vi "Robot Main.vi"() -> ()   [LabVIEW 2014]
doc: "This VI implements the framework and scheduler for your robotics program. It should not be necessary to modify the framework. You are expected to add your code to the VIs called from Robot Main - the ones located in the Team Code folder within the project."
uses:
  <vilib>/Rock Robotics/WPI/Camera/WPI_CameraImageSize.ctl
  Robot Global Data.vi
panel:
  out "Trace Buffer Size":i32
  in  "Image Size":T1=enum."320x240"
  in  "Enable Vision":bool
  in  "Finish":bool
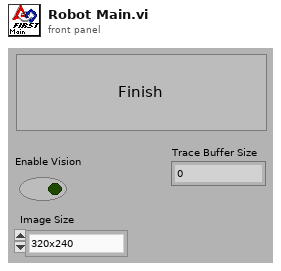
[diagram p1: front panel]
types:
  T1 = typedef "WPI_CameraImageSize.ctl" = enum16{"640x480", "320x240", "160x120", "Custom"}
  T2 = typedef "WPI_DriverStationMatch Info.ctl" = cluster{"Autonomous Elapsed Seconds":dbl, "TeleOp Elapsed Seconds":dbl, "Disabled Elapsed Seconds":dbl, "Visited Autonomous":bool, "Visited TeleOp":bool, "Visited Disabled":bool, "Autonomous Settings":cluster{"Autonomous Style":enum16{"Iterative", "Independent"}, "VI Refnum":refnum<vi>}}
  T3 = typedef "WPI_DriverStationDerivedRobotMode.ctl" = enum16{"Init", "Execute", "Stop"}
  T4 = typedef "WPI_DriverStationRobotMode2.ctl" = enum16{"Autonomous Disabled", "Autonomous Enabled", "Teleop Disabled", "Teleop Enabled", "Disconnected", "Finish", "Test Disabled", "Test Enabled", "Emergency Stopped"}
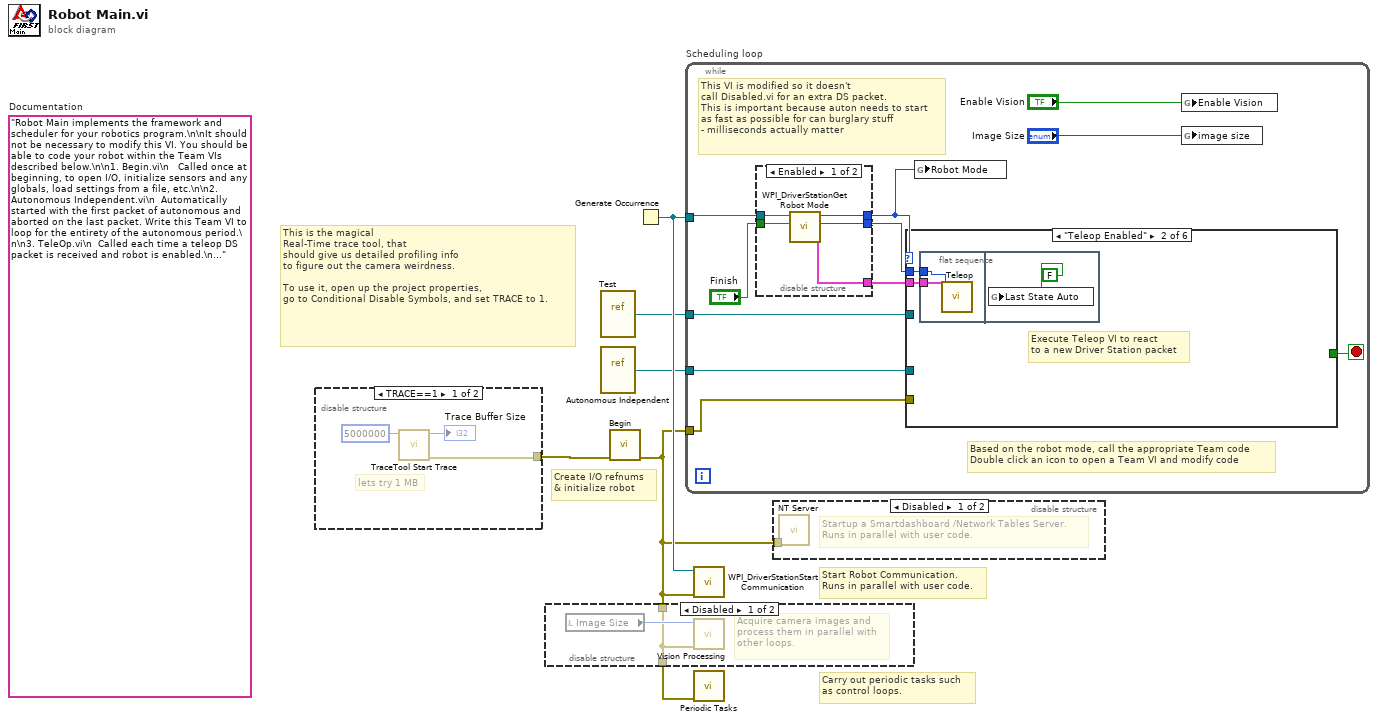
[diagram p0: block diagram]
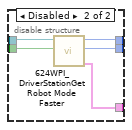
[diagram p5: hidden frame]
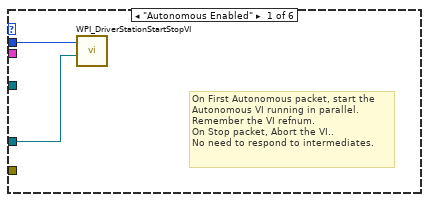
[diagram p6: hidden frame]
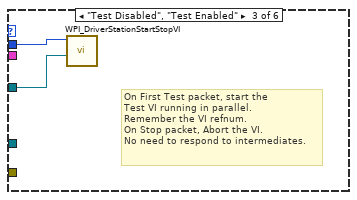
[diagram p7: hidden frame]
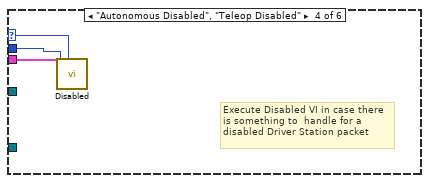
[diagram p8: hidden frame]
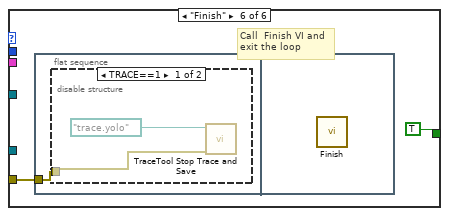
[diagram p10: hidden frame]
diagram:
  (unwired) "Robot Main implements the framework and scheduler for your robotics program.\n\nIt should not be necessary to modify this VI. You should be able to code your robot within the Team VIs described below.\n\n1. Begin.vi\n   Called once at beginning, to open I/O, initialize sensors and any globals, load settings from a file, etc.\n\n2. Autonomous Independent.vi\n  Automatically started with the first packet of autonomous and aborted on the last packet. Write this Team VI to loop for the entirety of the autonomous period.\n\n3. TeleOp.vi\n  Called each time a teleop DS packet is received and robot is enabled.\n\n4. Disabled.vi\n  Called each time a packet is received and the robot is disabled.\n\n5. Test.vi\n  Called Automatically started with the first test packet and aborted on the last. Modify this VI to carry out robot and sensor validation tests.\n\n6. Vision.vi\n  A parallel loop that acquires and processes camera images.\n\n7. PeriodicTasks.vi\n  Parallel loops running at user-defined rates.\n\n8. Finish.vi\n  Called before exiting, so you can save data, clean up I/O, etc.\n"  # Documentation
  # "Create I/O refnums\n& initialize robot"
  # "This is the magical\nReal-Time trace tool, that\nshould give us detailed profiling info \nto figure out the camera weirdness.\n\nTo use it, open up the project properties,\ngo to Conditional Disable Symbols, and set TRACE to 1."
  # "Carry out periodic tasks such\nas control loops."
  # "Start Robot Communication.\nRuns in parallel with user code."
  n1 = disable-structure shown="TRACE==1" {
    disable-tunnel: [w9 _] -> w1
    frame condition #0 {
      # "lets try 1 MB"
      n2 = call <vilib>:"TraceTool Start Trace.vi"("Buffer Size (250000 bytes)"=5000000) -> ("error out"=w9:errorcluster, "Actual Buffer Size"=→"Trace Buffer Size":i32)  [unwired: 9 in]
    }
    frame condition #1 (active) {
    }
  }
  n3 = vi-ref "Test.vi"() -> (w4:refnum<vi>)
  n4 = vi-ref "Autonomous Independent.vi"() -> (w5:refnum<vi>)
  n5 = call "Begin.vi"("error in"=w1) -> ("error out"=w2:errorcluster)  [unwired: 1 in, 9 out]
  n6 = disable-structure shown="Disabled" {
    disable-tunnel: w2 -> [w10 w12]
    disable-tunnel: [w10 w12] -> w3
    frame Disabled {
      # "Acquire camera images and\nprocess them in parallel with\nother loops."
      n7 = local read "Image Size"() -> (w11:T1)
      n8 = call "Vision Processing.vi"("error in (no error)"=w10, "Image Size"=w11) -> ()  [unwired: 6 out]
    }
    frame Enabled {
    }
  }
  n9 = Generate Occurrence() -> (w6:refnum<k4>)
  n10 = while "Scheduling loop" {
    tunnel: w6 -> [w22]
    tunnel: w5 -> [w17]
    tunnel: w4 -> [w15]
    tunnel: w2 -> [w13]
    stop <- w19 stop-if-true
    # "This VI is modified so it doesn't\ncall Disabled.vi for an extra DS packet.\nThis is important because auton needs to start\nas fast as possible for can burglary stuff \n- milliseconds actually matter"
    # "Based on the robot mode, call the appropriate Team code\nDouble click an icon to open a Team VI and modify code"
    n11 = disable-structure shown="Enabled" {
      disable-tunnel: [w28 w30] -> w23
      disable-tunnel: w22 -> [w27 w33]
      disable-tunnel: "Finish" -> [w26 w32]
      disable-tunnel: [w25 w29] -> w20
      disable-tunnel: [w24 w31] -> w14
      frame Enabled {
        n12 = call <vilib>:"WPI_DriverStationGet Robot Mode.vi"("Finish"=w26, "DS Occurrence"=w27) -> ("Match Info out"=w25:T2, "Call Context"=w28:T3, "Robot Mode"=w24:T4)  [unwired: 7 out]
      }
      frame Disabled {
        n13 = call "624WPI_DriverStationGet Robot Mode Faster.vi"("Finish"=w32, "DS Occurrence"=w33) -> ("Match Info out"=w29:T2, "Call Context"=w30:T3, "Robot Mode"=w31:T4)  [unwired: 6 in, 1 out]
      }
    }
    n14 = case shown="\"Teleop Enabled\"" w14 {
      selector: w14 -> [_ _ _ w43 _ _]
      tunnel: w23 -> [w35 w37 w42 w45 _ _]
      tunnel: w20 -> [_ w36 _ w44 _ _]
      tunnel: [_ _ _ _ _ TRUE] -> w19
      tunnel: w17 -> [w34 _ _ _ _ _]
      tunnel: w15 -> [_ _ w41 _ _ _]
      tunnel: w13 -> [_ _ _ _ _ w46]
      frame "Autonomous Enabled" {
        # "On First Autonomous packet, start the\nAutonomous VI running in parallel.\nRemember the VI refnum.\nOn Stop packet, Abort the VI..\nNo need to respond to intermediates."
        n15 = call <vilib>:"WPI_DriverStationStartStopVI.vi"("VI in"=w34, "Call Context"=w35) -> ()  [unwired: 10 in]
      }
      frame "Teleop Enabled" {
        # "Execute Teleop VI to react\nto a new Driver Station packet"
        n16 = flat-sequence {
          tunnel: w37 -> [w39]
          tunnel: w36 -> [w38]
          frame #0 {
            n17 = call "Teleop.vi"("Match Info"=w38, "Call Context"=w39) -> ()  [unwired: 1 in, 9 out]
          }
          frame #1 {
            n18 = global write "Robot Global Data.vi" "Last State Auto"(FALSE ("Last State Auto")) -> ()
          }
        }
      }
      frame "Test Disabled", "Test Enabled" {
        # "On First Test packet, start the\nTest VI running in parallel.\nRemember the VI refnum.\nOn Stop packet, Abort the VI.\nNo need to respond to intermediates."
        n19 = call <vilib>:"WPI_DriverStationStartStopVI.vi"("VI in"=w41, "Call Context"=w42) -> ()  [unwired: 10 in]
      }
      frame "Autonomous Disabled", "Teleop Disabled" {
        # "Execute Disabled VI in case there\nis something to  handle for a\ndisabled Driver Station packet"
        n20 = call "Disabled.vi"("Robot Mode"=w43, "Match Info"=w44, "Call Context"=w45) -> ()  [unwired: 1 in, 8 out]
      }
      frame "Disconnected", Default {
        # "Driver Station packet didn't arrive.\nPossibly useful for diagnostics"
      }
      frame "Finish" {
        # "Call  Finish VI and\nexit the loop"
        n21 = flat-sequence {
          tunnel: w46 -> [w48]
          frame #0 {
            n22 = disable-structure shown="TRACE==1" {
              disable-tunnel: w48 -> [w49 _]
              frame condition #0 {
                n23 = call <vilib>:"TraceTool Stop Trace and Save.vi"("error in (no error)"=w49, "Path to Trace Log"=path "/trace.yolo") -> ()  [unwired: 9 in, 1 out]
              }
              frame condition #1 (active) {
              }
            }
          }
          frame #1 {
            n24 = call "Finish.vi"() -> ()  [unwired: 1 in, 7 out]
          }
        }
      }
    }
    n25 = global write "Robot Global Data.vi" "Robot Mode"(w14) -> ()
    n26 = global write "Robot Global Data.vi" "Enable Vision"("Enable Vision") -> ()
    n27 = global write "Robot Global Data.vi" "image size"("Image Size") -> ()
  }
  n28 = call <vilib>:"WPI_DriverStationStart Communication.vi"("error in (no error)"=w2, "occurrence"=w6) -> ()  [unwired: 10 out]
  n29 = call "Periodic Tasks.vi"("error in (no error)"=w3) -> ()  [unwired: 1 in, 10 out]
  n30 = disable-structure shown="Disabled" {
    disable-tunnel: w2 -> [w51 _]
    frame Disabled {
      # "Startup a Smartdashboard /Network Tables Server.\nRuns in parallel with user code."
      n31 = call <vilib>:"NT Server.vi"("error in (no error)"=w51) -> ()  [unwired: 11 in]
    }
    frame Enabled {
    }
  }
